vi "_Beep_Done.vi"(4 "状态输入":bool) -> (1 "状态输出":bool)   [LabVIEW 2020, in "Beep.lvlib"]
uses:
  Beep.lvlib
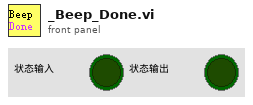
[diagram p1: front panel]
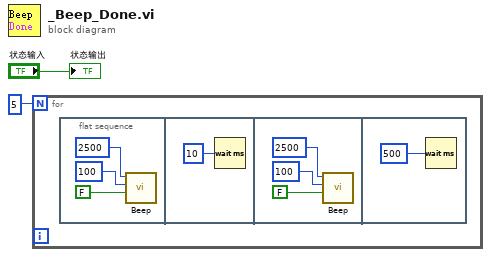
[diagram p0: block diagram]
diagram:
  n1 = for {
    N: 5 -> [_]
    n2 = flat-sequence {
      frame #0 {
        n3 = call <vilib>:"Beep.vi"("use system alert? (T)"=FALSE, "duration (msec)"=100, "frequency (Hz)"=2500) -> ()  [unwired: 9 in]
      }
      frame #1 {
        n4 = Wait (ms)(milliseconds to wait=10) -> ()  [unwired: 1 out]
      }
      frame #2 {
        n5 = call <vilib>:"Beep.vi"("use system alert? (T)"=FALSE, "duration (msec)"=100, "frequency (Hz)"=2500) -> ()  [unwired: 9 in]
      }
      frame #3 {
        n6 = Wait (ms)(milliseconds to wait=500) -> ()  [unwired: 1 out]
      }
    }
  }
  "状态输出" <- "状态输入"
